vi "Prop Valve Fast Forward.vi"(5 "Init":bool, 7 "Direction":T1=enum."DUT", 8 "error in (no error)":errorcluster, 11 "Stand in":refnum<class "Stand.lvclass">) -> (0 "error out":errorcluster, 2 "Done":bool caption="Time has Elapsed")   [LabVIEW 2019, in "Stand.lvclass"]
uses:
  Stand.lvclass
  C:/Users/ANENKOV_V1/Desktop/src/Device_class/Device.lvclass
  TypeDef/Direction.ctl
  Device_class/Device.lvclass/Device.ctl
  Stand.lvclass/Stand.ctl
  AI_class/AI.lvclass/AI.ctl
  AnalogComparator_class/AnalogComparator.lvclass/AnalogComparator.ctl
  OscillationClass/OscillationDetector.lvclass/OscillationDetector.ctl
  AnalogComparator_class/GetStatus.vi
  OscillationClass/Read DATA.vi
  FPGA_API_class/FPGA API.lvclass
  Device_class/Device.lvclass
  AI_class/AI.lvclass
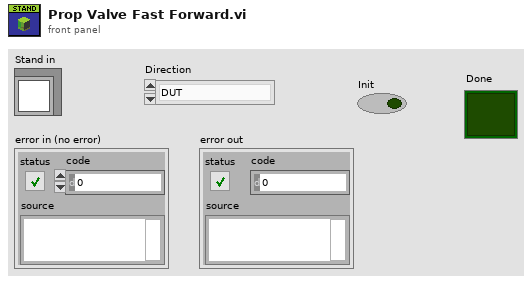
[diagram p1: front panel]
types:
  T1 = typedef "Direction.ctl" = enum16{"None", "DUT", "Chamber"}
  T2 = typedef "AI_Data.ctl" = cluster{"Stat Data":T3, "OutOfRangeMax":bool, "OutOfRangeMin":bool, "HIHI":bool, "HI":bool, "LO":bool, "LOLO":bool, "DATA N":T4, "DATA PERIOD":T4, "UPPER TH":dbl, "LOWER TH":dbl}
  T3 = typedef "AI Statistics Data.ctl" = cluster{"raw mean":dbl, "scl mean":dbl, "raw mean 1Hz":dbl, "scl mean 1Hz":dbl}
  T4 = typedef "DATA Oscill.ctl" = cluster{"SUM":dbl, "COUNTER":dbl, "MAX CURR":dbl, "MIN CURR":dbl, "AVR":dbl, "MAX":dbl, "MIN":dbl, "DELTA AVR":dbl, "DELTA MAX":dbl, "DELTA MIN":dbl, "PERIOD":dbl}
  T5 = typedef "Setting Pressure PI.ctl" = cluster{"P [MPa]":dbl, "A [MPa/V]":dbl, "P0 [MPa]":dbl, "P start [%]":dbl, "P end [%]":dbl, "T0 DUT [s]":dbl, "T0 CMBR [s]":dbl}
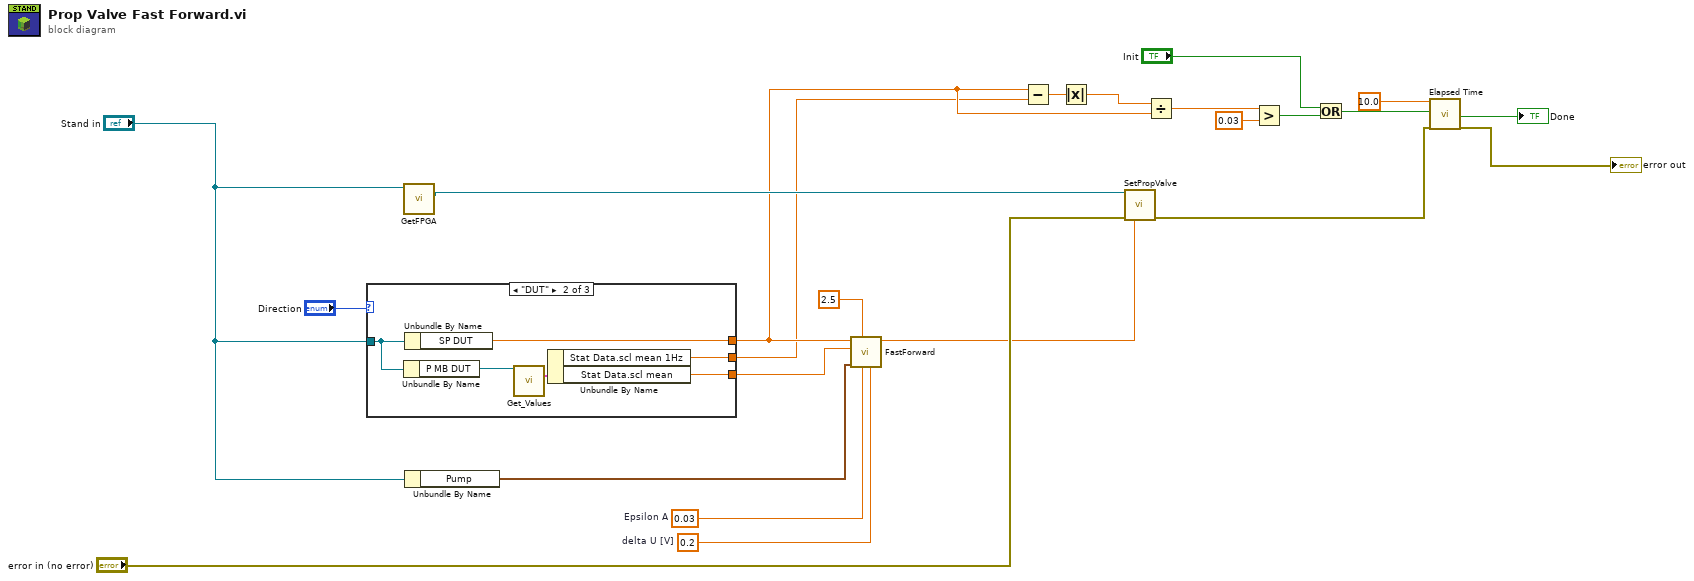
[diagram p0: block diagram]
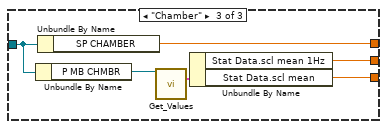
[diagram p3: hidden frame]
diagram:
  w22 = 0.2  # delta U [V]
  w21 = 0.03  # Epsilon A
  n1 = case shown="\"DUT\"" "Direction" {
    tunnel: [_ w29 w35] -> w4
    tunnel: [_ w27 w33] -> w5
    tunnel: "Stand in" -> [_ w26 w32]
    tunnel: [_ w24 w30] -> w1
    frame "None", Default {
    }
    frame "DUT" {
      n2 = Unbundle By Name(w26) -> ("P MB DUT"=w25:refnum<class "AI.lvclass">)
      n3 = Unbundle By Name(w26) -> ("SP DUT"=w27:dbl)
      n4 = call "Get_Values.vi"("reference in"=w25) -> ("Data"=w28:T2)  [unwired: 14 in]
      n5 = Unbundle By Name(w28) -> ("Stat Data.scl mean 1Hz"=w24:dbl, "Stat Data.scl mean"=w29:dbl)
    }
    frame "Chamber" {
      n6 = Unbundle By Name(w32) -> ("P MB CHMBR"=w31:refnum<class "AI.lvclass">)
      n7 = Unbundle By Name(w32) -> ("SP CHAMBER"=w33:dbl)
      n8 = call "Get_Values.vi"("reference in"=w31) -> ("Data"=w34:T2)  [unwired: 14 in]
      n9 = Unbundle By Name(w34) -> ("Stat Data.scl mean 1Hz"=w30:dbl, "Stat Data.scl mean"=w35:dbl)
    }
  }
  n10 = call "GetFPGA.vi"("Device in"="Stand in") -> ("FPGA API.lvclass"=w18:refnum<class "FPGA API.lvclass">)  [unwired: 10 in]
  n11 = Unbundle By Name("Stand in") -> ("Pump"=w17:T5)
  n12 = call "FastForward.vi"("delta U [V]"=w22, "Epsilon A"=w21, "U min [V]"=2.5, "Setting"=w17, "PV"=w4, "SP"=w5) -> ("U"=w19:dbl)  [unwired: 5 in]
  n13 = Subtract(x=w5, y=w1) -> (x-y=w14:dbl)
  n14 = Absolute Value(x=w14) -> (abs(x)=w13:dbl)
  n15 = call-dynamic "SetPropValve.vi"("FPGA API in"=w18, "error in (no error)"="error in (no error)", "AO 1"=w19) -> ("error out"=w3:errorcluster)  [unwired: 11 in, 1 out]
  n16 = Divide(x=w13, y=w5) -> (x/y=w12:dbl)
  n17 = Greater?(x=w12, y=0.03) -> (0:w10:bool)
  n18 = Or(x="Init", y=w10) -> (x .or. y?=w9:bool)
  n19 = call "Elapsed Time"("Time Target (s)"=10.0, "Reset"=w9, "error in (no error)"=w3) -> ("Time has Elapsed"=→"Done":bool, "error out"=→"error out":errorcluster)  [unwired: 9 in, 6 out]
